vi "FindFromINI.vi"(8 "error in (no error)":errorcluster, 11 "INI folder":path) -> (0 "error out":errorcluster, 1 "IDs":u32[](array[numeric]), 2 "Families":u32[](array[numeric]), 3 "Names":string[](array[string]))   [LabVIEW 2019, in "LINXx.lvlib"]
uses:
  LINXx.lvlib
  <vilib>/regexp/Match Regular Expression.xnode
  <vilib>/Utility/config.llb/NI_LVConfig.lvlib
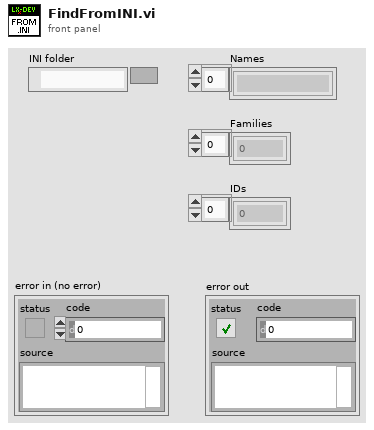
[diagram p1: front panel]
types:
  T1 = typedef "NI_LVConfig.lvlib/Config Data RefNum.ctl" = refnum<k1>
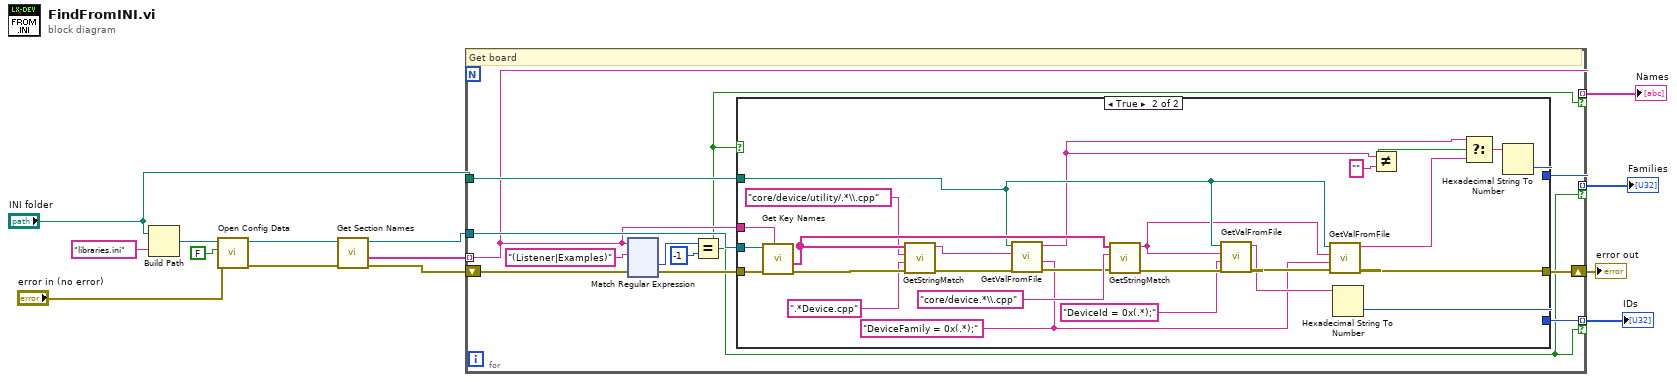
[diagram p0: block diagram]
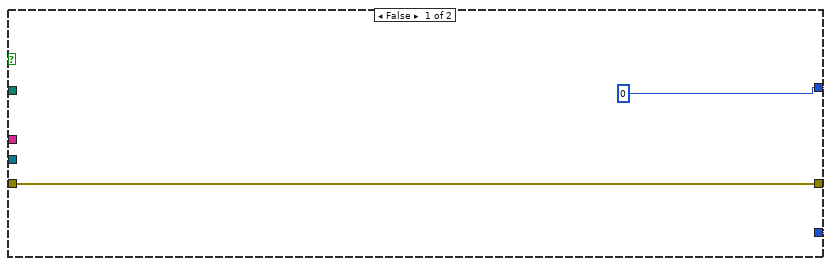
[diagram p2: hidden frame]
diagram:
  n1 = Build Path(base path="INI folder", name or relative path="libraries.ini") -> (appended path=w5:path)
  n2 = call <vilib>:"Open Config Data.vi"("error in (no error)"="error in (no error)", "create file if necessary (T)"=FALSE, "configuration file path"=w5) -> ("error out"=w6:errorcluster, "refnum"=w7:T1)  [unwired: 6 in, 1 out]
  n3 = call <vilib>:"Get Section Names.vi"("error in (no error)"=w6, "refnum"=w7) -> ("error out"=w9:errorcluster, "section names"=w10:string[], "refnum out"=w8:T1)  [unwired: 7 in]
  n4 = for {
    tunnel: w8 -> [w23]
    tunnel: w10 -> [w16] mode=indexing
    shift-right: [w21] -> w1
    shift-left: w9 -> [w24]
    tunnel: "INI folder" -> [w22]
    tunnel: [w18] -> w13 mode=indexing if=w15
    tunnel: [w17] -> w14 mode=indexing if=w15
    tunnel: [w16] -> w12 mode=indexing if=w15
    # "Get board"
    n5 = xnode "Match Regular Expression"("input string"=w16, "regular expression"="(Listener|Examples)", "error in"=w24) -> ("offset past match"=w20:i32, "error out"=w25:errorcluster)  [unwired: 3 in, 3 out]
    n6 = Equal?(x=w20, y=-1) -> (x = y?=w15:bool)
    n7 = case shown="True" w15 {
      tunnel: w16 -> [_ w41]
      tunnel: w25 -> [w28 w54]
      tunnel: w23 -> [_ w53]
      tunnel: w22 -> [_ w38]
      tunnel: [w28 w39] -> w21
      tunnel: [w27 w31] -> w18
      tunnel: [w27 w30] -> w17
      frame False {
        w27 = u32 0
      }
      frame True {
        w29 = "DeviceFamily = 0x(.*);" ("regular expression")
        n8 = call <vilib>:"Get Key Names.vi"("section"=w41, "error in (no error)"=w54, "refnum"=w53) -> ("error out"=w45:errorcluster, "key names"=w51:string[])  [unwired: 5 in, 2 out]
        n9 = call "GetStringMatch.vi"("error in (no error)"=w45, "Reject Regex"=".*Device.cpp", "Match Regex"="core/device/utility/.*\\.cpp" ("Regex"), "String"=w51) -> ("error out"=w49:errorcluster, "Matching string"=w48:string)  [unwired: 6 in]
        n10 = call "GetValFromFile.vi"("error in (no error)"=w49, "regular expression"=w29, "File path"=w48, "FW path"=w38) -> ("error out"=w44:errorcluster, "extracted value"=w33:string)  [unwired: 6 in]
        n11 = call "GetStringMatch.vi"("error in (no error)"=w44, "Match Regex"="core/device.*\\.cpp" ("regular expression"), "String"=w51) -> ("error out"=w47:errorcluster, "Matching string"=w37:string)  [unwired: 7 in]
        n12 = call "GetValFromFile.vi"("error in (no error)"=w47, "regular expression"="DeviceId = 0x(.*);", "File path"=w37, "FW path"=w38) -> ("error out"=w40:errorcluster, "extracted value"=w42:string)  [unwired: 6 in]
        n13 = call "GetValFromFile.vi"("error in (no error)"=w40, "regular expression"=w29, "File path"=w37, "FW path"=w38) -> ("error out"=w39:errorcluster, "extracted value"=w35:string)  [unwired: 6 in]
        n14 = Hexadecimal String To Number(string=w42) -> (number=w30:u32)  [unwired: 2 in, 1 out]
        n15 = Not Equal?(x=w33, y="") -> (x != y?=w34:bool)
        n16 = Select(t=w33, s=w34, f=w35) -> (s? t:f=w36:string)
        n17 = Hexadecimal String To Number(string=w36) -> (number=w31:u32)  [unwired: 2 in, 1 out]
      }
    }
  }
  "IDs" <- w14
  "Families" <- w13
  "Names" <- w12
  "error out" <- w1
